vi "Write V2 Trigger Settings.vi"(8 "error in (no error)":errorcluster, 10 "V2 Trigger Settings":T1={"Gate Type"=TRUE, "Synchronize Gate"=FALSE, "Force Trigger (µs)"=0.0, "MS Bus"=1} {"MS Bus" format="%04x" items=["Local Primary"=1, "Local Secondary"=2, "Local Force"=4, "Resynchronize"=8, "Master Primary"=16, "Master Secondary"=32, "Master Force"=64, "System Clock"=128, "Delay Clock"=256, "Inhibit Local"=512, "Start Local"=1024, "Start Bus"=2048, "Step Back Local"=4096, "Step Back Bus"=8192, "Enable From E"=65536, "Enable From F"=131072, "Enable From Bus"=262144]; "Force Trigger (µs)" min=0.0 format="%.6f"}, 11 "BME_DG_G05 in":refnum<class "BME_DG_G05.lvclass">) -> (0 "error out":errorcluster, 3 "BME_DG_G05 out":refnum<class "BME_DG_G05.lvclass">)   [LabVIEW 2009, in "BME_DG_G05.lvclass"]
uses:
  BME_DG_G05.lvclass
  BME_DG_G05.lvclass/BME_DG_G05.ctl
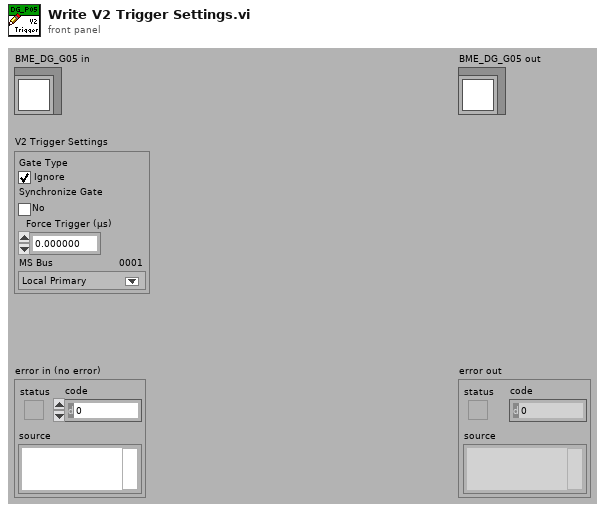
[diagram p1: front panel]
types:
  T1 = cluster{"Gate Type":bool, "Synchronize Gate":bool, "Force Trigger (µs)":dbl, "MS Bus":u32}
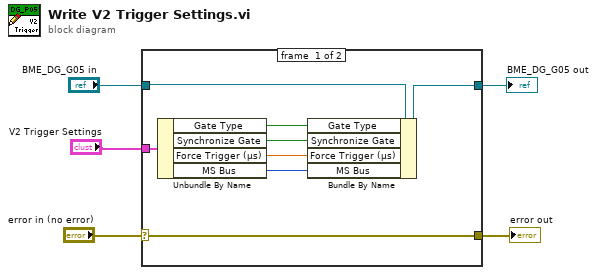
[diagram p0: block diagram]
diagram:
  n1 = case shown="No Error" "error in (no error)" {
    selector: "error in (no error)" -> [w6 w15]
    tunnel: "V2 Trigger Settings" -> [w13 _]
    tunnel: [w8 w14] -> w4
    tunnel: "BME_DG_G05 in" -> [w7 w14]
    tunnel: [w6 w15] -> w1
    frame #0 {
      n2 = Unbundle By Name(w13) -> ("Gate Type"=w12:bool, "Synchronize Gate"=w10:bool, "Force Trigger (µs)"=w9:dbl, "MS Bus"=w11:u32)
      n3 = Bundle By Name(cluster=w7, "Gate Type"=w12, "Synchronize Gate"=w10, "Force Trigger (µs)"=w9, "MS Bus"=w11) -> (w8:refnum<class "BME_DG_G05.lvclass">)
    }
    frame #1 {
    }
  }
  "error out" <- w1
  "BME_DG_G05 out" <- w4
